vi "Acquire Mapped Memory Access.vi"   [LabVIEW 2020, in "image.lvlib"]
doc: "Get direct access to a pointer to the underlying image memory - this is useful for integration with other external libraries which expect a pointer to a memory loctation.\n\nThis VI locks the image into \"mapped access mode\" and provides a Data Value Reference which can be used with an in-place-element structure to get memory address and layout information.\n\nThe image can be unlocked by calling \"Release Mapped Memory Access.vi\""
uses:
  image.lvlib
  Mapped Memory Access Image ARGB/Mapped Memory Access Image ARGB.lvclass
  Mapped Memory Access Image Greyscale/Mapped Memory Access Image Greyscale.lvclass
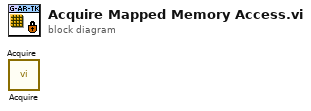
[diagram p0: block diagram]
diagram:
  n1 = call "Acquire.vi"() -> ()  [unwired: 10 in, 2 out]
  n2 = call "Acquire.vi"() -> ()  [unwired: 10 in, 2 out]
